vi "Set Assert VI Name.vi"(7 "VI Path":path, 8 "error in (no error)":errorcluster, 11 "Test in":refnum<class "Test.lvclass">) -> (0 "error out":errorcluster, 3 "Test out":refnum<class "Test.lvclass">)   [LabVIEW 2018, in "Test.lvclass"]
uses:
  Test.lvclass
  Test Class String IDs.vi
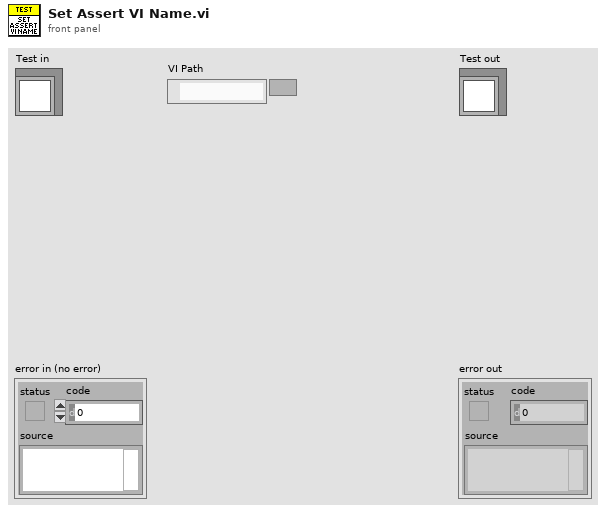
[diagram p1: front panel]
types:
  T1 = cluster{"Comparison Value 1":string, "Comparison Value 2":string, "Invert Result":string, "Assert VI Name":string, "Data Type":string, "Builder User Name":string, "Build Timestamp":string, "Failure Action":string, "Comment":string, "Assert Name":string, "Description":string, "Evaluation String":string, "MD5":string}
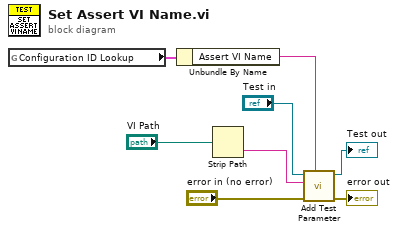
[diagram p0: block diagram]
diagram:
  n1 = global read "Test Class String IDs.vi" "Configuration ID Lookup"() -> (w2:T1)
  n2 = Unbundle By Name(w2) -> ("Assert VI Name"=w1:string)
  n3 = Strip Path(path="VI Path") -> (name=w3:string)  [unwired: 1 out]
  n4 = call-dynamic "Add Test Parameter.vi"("Data Value ID"=w1, "error in (no error)"="error in (no error)", "Data Value"=w3, "Test in"="Test in") -> ("error out"=→"error out":errorcluster, "Test out"=→"Test out":refnum<class "Test.lvclass">)  [unwired: 5 in, 1 out]
